vi "queue_array_back.vi"(8 "error in":errorcluster, 10 "array":string[](array[string])=["Data: Initialize", "Initialize Core Data", "Data: Get Case Strings", "Data: Get Case Documentation", "UI: Initialize", "UI: Front Panel State >> Open", "Delay >> 1000"], 11 "queue in":refnum<queue>) -> (0 "error out":errorcluster, 3 "queue out":refnum<queue>)   [LabVIEW 2012]
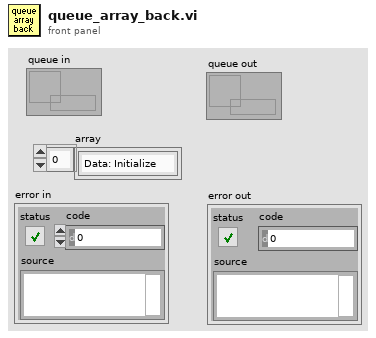
[diagram p1: front panel]
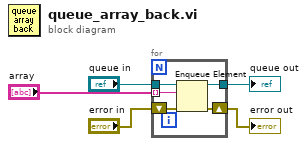
[diagram p0: block diagram]
diagram:
  n1 = for {
    tunnel: [w10] -> w5
    tunnel: "queue in" -> [w9]
    shift-right: [w7] -> w4
    shift-left: "error in" -> [w8]
    tunnel: "array" -> [w6] mode=indexing
    n2 = Enqueue Element(queue=w9, element=w6, error in (no error)=w8) -> (queue out=w10:refnum<queue>, error out=w7:errorcluster)  [unwired: 1 in, 1 out]
  }
  "queue out" <- w5
  "error out" <- w4
